vi "Extract All Files to Directory.vi"(8 "error in (no error)":errorcluster, 10 "Extract to Dir":path, 11 "Zip File Path":path) -> (0 "error out":errorcluster)   [LabVIEW 2019, in "Command-Line Zip.lvlib"]
uses:
  <userlib>/_OpenG.lib/file/file.llb/Strip Path Extension - String__ogtk.vi
  Command-Line Zip.lvlib
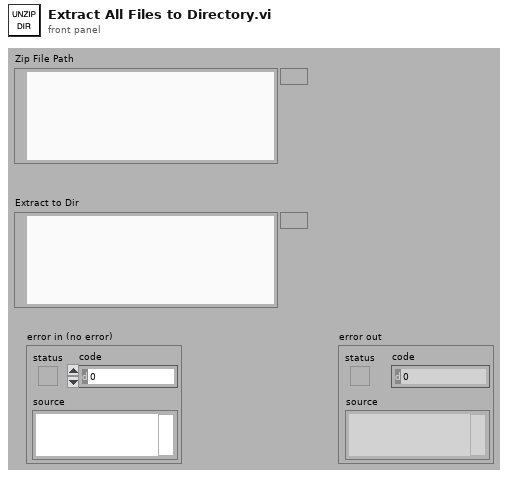
[diagram p1: front panel]
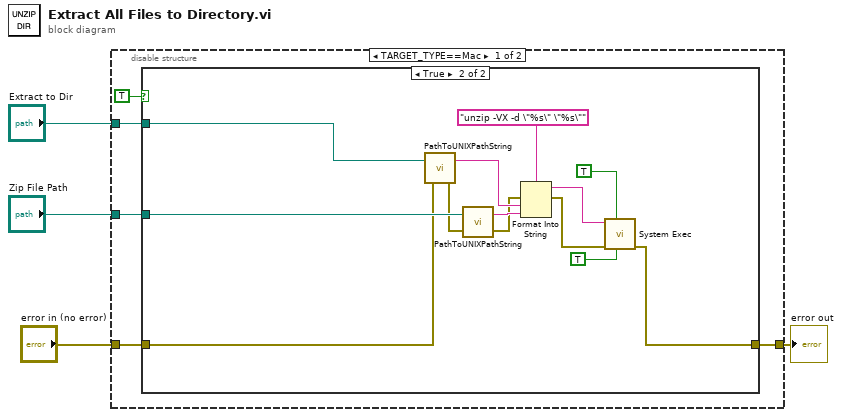
[diagram p0: block diagram]
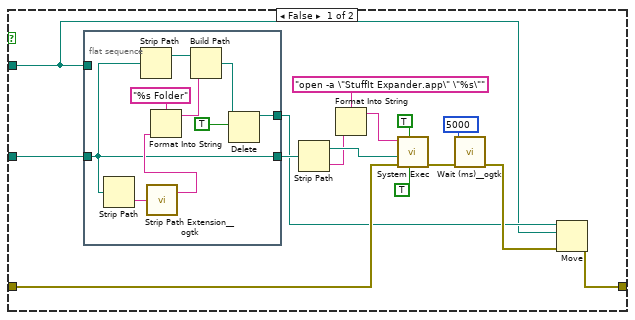
[diagram p2: hidden frame]
diagram:
  n1 = disable-structure shown="TARGET_TYPE==Mac" {
    disable-tunnel: "Zip File Path" -> [w9 _]
    disable-tunnel: "Extract to Dir" -> [w8 _]
    disable-tunnel: "error in (no error)" -> [w7 w47]
    disable-tunnel: [w6 w47] -> w1
    frame condition #0 (active) {
      n2 = case shown="True" TRUE {
        tunnel: w9 -> [w20 w45]
        tunnel: w8 -> [w10 w43]
        tunnel: w7 -> [w18 w38]
        tunnel: [w12 w37] -> w6
        frame False {
          n3 = flat-sequence {
            tunnel: w20 -> [w26]
            tunnel: w10 -> [_]
            tunnel: [w26] -> w17
            tunnel: [w30] -> w11
            frame #0 {
              n4 = Strip Path(path=w26) -> (name=w25:string)  [unwired: 1 out]
              n5 = Strip Path(path=w26) -> (stripped path=w33:path)  [unwired: 1 out]
              n6 = call-poly <userlib>:"Strip Path Extension__ogtk.vi"("path"=w25) -> ("root"=w29:string)  [unwired: 1 out]
              n7 = Format Into String(format string="%s Folder", w29) -> (resulting string=w27:string)  [unwired: 2 in, 1 out]
              n8 = Build Path(base path=w33, name or relative path=w27) -> (appended path=w32:path)
              n9 = Delete(path (use dialog)=w32, entire hierarchy (F)=TRUE) -> (deleted path=w30:path)  [unwired: 3 in, 2 out]
            }
          }
          n10 = Strip Path(path=w17) -> (stripped path=w16:path, name=w15:string)
          n11 = Format Into String(format string="open -a \"StuffIt Expander.app\" \"%s\"" ("command line"), w15) -> (resulting string=w13:string)  [unwired: 2 in, 1 out]
          n12 = call <vilib>:"System Exec.vi"("run minimized? (F)"=TRUE, "wait until completion? (T)"=TRUE, "error in (no error)"=w18, "working directory"=w16, "command line"=w13) -> ("error out"=w21:errorcluster)  [unwired: 3 in, 3 out]
          n13 = call <userlib>:"Wait (ms)__ogtk.vi"("error in (no error)"=w21, "milliseconds to wait"=u32 5000) -> ("error out"=w19:errorcluster)  [unwired: 8 in, 1 out]
          n14 = Move(source path=w11, error in=w19, 10:w10) -> (error out=w12:errorcluster)  [unwired: 2 in, 2 out]
        }
        frame True {
          n15 = call <vilib>:"PathToUNIXPathString.vi"("error in (no error)"=w38, "LV Path"=w43) -> ("error out"=w41:errorcluster, "UNIX Path"=w42:string)
          n16 = call <vilib>:"PathToUNIXPathString.vi"("error in (no error)"=w41, "LV Path"=w45) -> ("error out"=w40:errorcluster, "UNIX Path"=w44:string)
          n17 = Format Into String(format string="unzip -VX -d \"%s\" \"%s\"", error in=w40, w42, w44) -> (resulting string=w36:string, error out=w39:errorcluster)  [unwired: 1 in]
          n18 = call <vilib>:"System Exec.vi"("run minimized? (F)"=TRUE, "wait until completion? (T)"=TRUE, "error in (no error)"=w39, "command line"=w36) -> ("error out"=w37:errorcluster)  [unwired: 4 in, 3 out]
        }
      }
    }
    frame condition #1 {
    }
  }
  "error out" <- w1
